vi "Read TDMS.vi"(8 "error in (no error)":errorcluster, 11 "file path":path=path "C:/Users/KT Chiam/Downloads/tdk tdms/AI Data_2021_Nov_20_17_10_07.tdms") -> (0 "error out":errorcluster, 3 "Waveform Graph":waveform(dbl)[](graph))   [LabVIEW 2019]
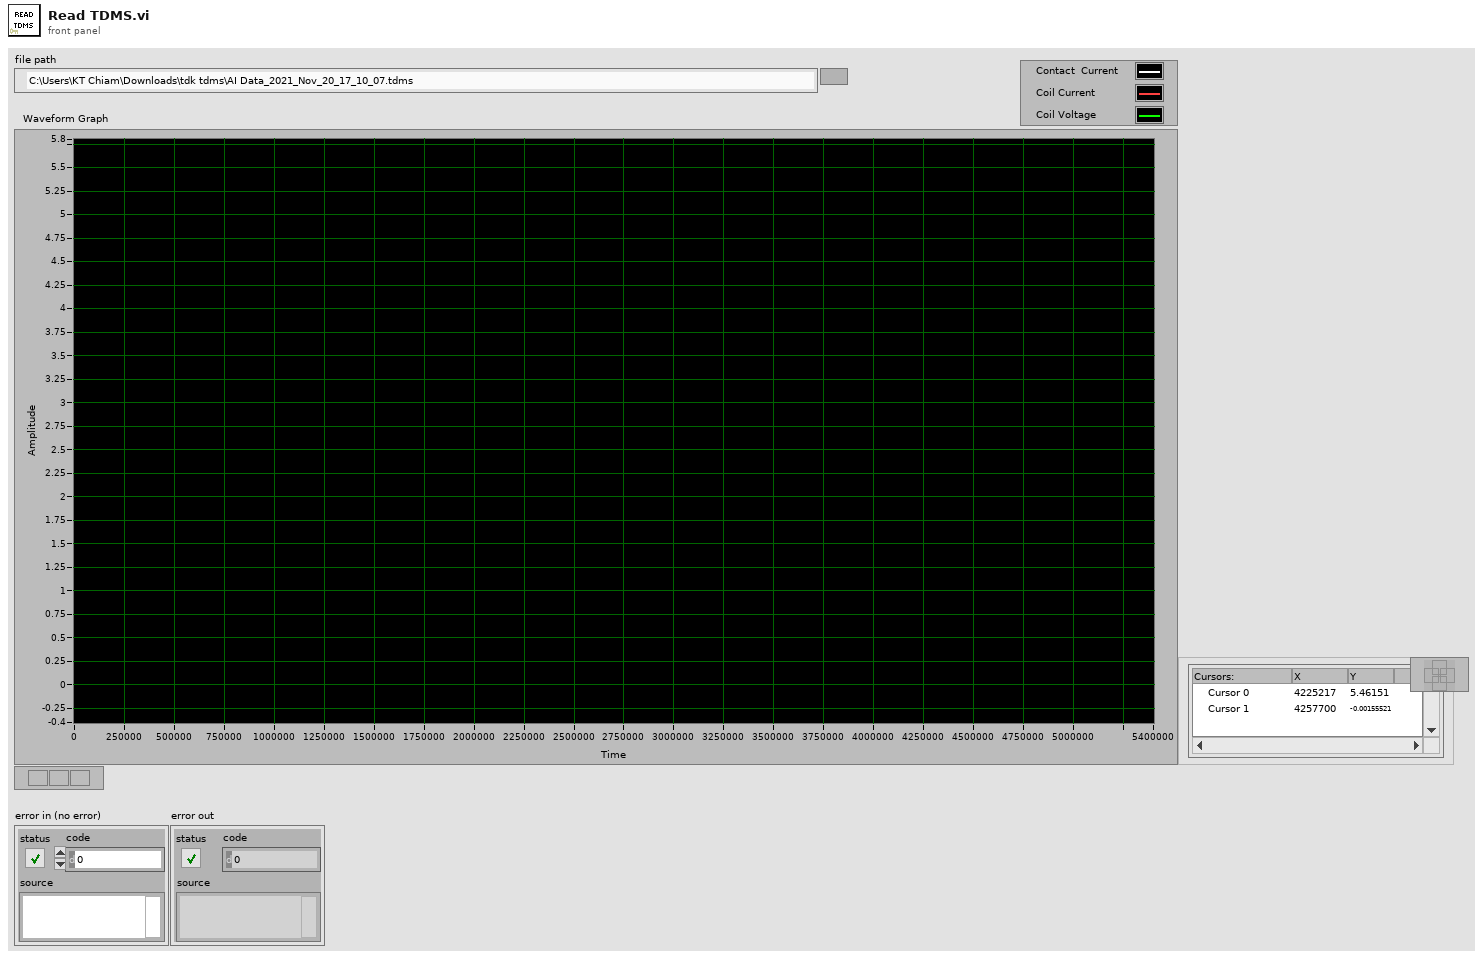
[diagram p1: front panel]
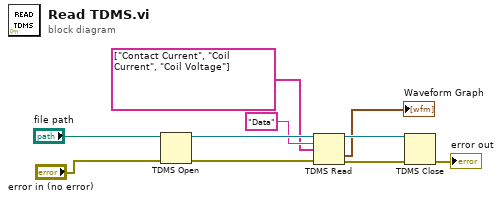
[diagram p0: block diagram]
diagram:
  n1 = TDMS Open(8:"error in (no error)", 11:"file path") -> (0:w3:errorcluster, 3:w9:refnum<k34>)  [unwired: 5 in]
  n2 = TDMS Read(0:w9, 5:"Data" ("group name in"), 7:string[] ["Contact Current", "Coil Current", "Coil Voltage"] ("channel name(s) in"), 11:w3) -> (4:w6:refnum<k34>, 10:→"Waveform Graph":waveform(dbl)[], 15:w2:errorcluster)  [unwired: 4 in, 3 out]
  n3 = TDMS Close(8:w2, 11:w6) -> (0:→"error out":errorcluster)  [unwired: 1 out]
